vi "Global tdms reference.vi"() -> ()   [LabVIEW 2016]
doc: "-----------------------------------------------------------------------------------------------------------------------\nCopyright <2019> <The University of Tennessee at Knoxville and the University of Tennessee Research Foundation>\nThis software is released under BSD-3 \nhttps://opensource.org/licenses/BSD-3-Clause \nAdditional license options available at https://utrf.tennessee.edu/industry/sample-agreements/\n-----------------------------------------------------------------------------------------------------------------------"
panel:
  out "PV tdms file out":refnum<k34>
  out "Switch tdms file out":refnum<k34>
  out "Batt tdms file out":refnum<k34>
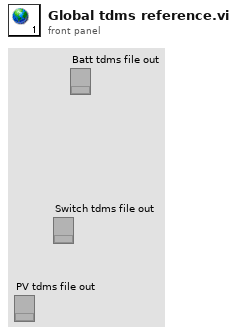
[diagram p1: front panel]
diagram:
